vi "ListboxStimulus.vi"(11 "error in (no error)":errorcluster) -> (15 "error out":errorcluster)   [LabVIEW 2016, in "DronaTest.lvlib"]
uses:
  DronaTest.lvlib
  APIs/Stimulus/ControlValue/SetValueAuto.vi
  APIs/Stimulus/ControlValue/Controls/Listbox/SetValueByItemIndex.vi
  APIs/Assert/AssertControlValue/Equal.vi
  APIs/Stimulus/ControlValue/Controls/Listbox/SetValueByItemName.vi
  APIs/Stimulus/VI/CloseVI.vi
  <vilib>/addons/_JKI Toolkits/Caraya/classes/Test/Test.lvclass
  Drona.lvlib
  <vilib>/SLL Toolkit/SLL Debug/SLL Debug.lvlib
  APIs/Stimulus/ControlValue/ControlValue.lvlib
  APIs/Assert/AssertControlValue/AssertControlValue.lvlib
  APIs/Stimulus/VI/VI.lvlib
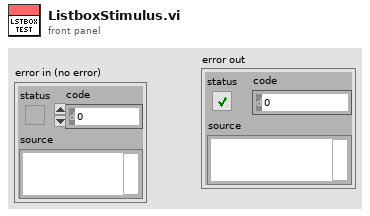
[diagram p1: front panel]
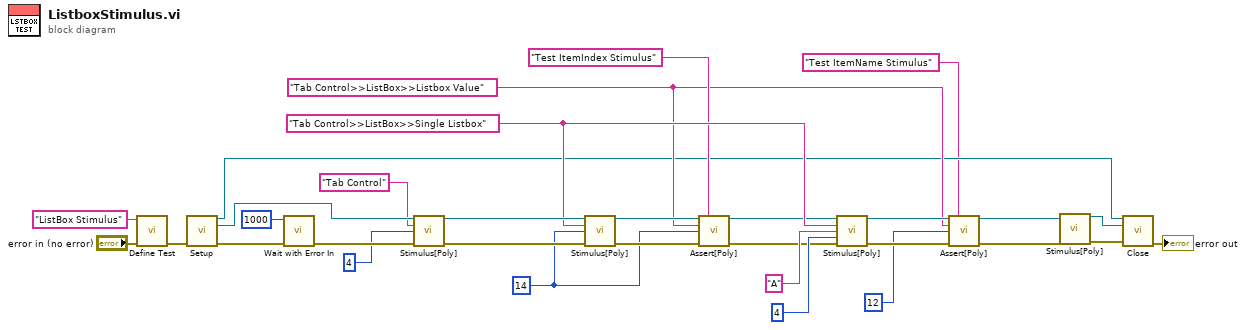
[diagram p0: block diagram]
diagram:
  w8 = "Tab Control>>ListBox>>Listbox Value" ("Control Path")
  w14 = 14 ("Item Index")
  w17 = "Tab Control>>ListBox>>Single Listbox" ("Control Path")
  n1 = call <vilib>:"Define Test.vi"("error in (no error)"="error in (no error)", "Label (VI Title)"="ListBox Stimulus") -> ("error out"=w30:errorcluster)  [unwired: 9 in]
  n2 = call "Setup.vi"("error in"=w30) -> ("Application Ref"=w2:refnum<vi>, "VI Reference Out"=w24:refnum<vi>, "error out"=w29:errorcluster)  [unwired: 12 in]
  n3 = call <vilib>:"Wait with Error In.vi"("error in (no error)"=w29, "milliseconds to wait"=u32 1000) -> ("error out"=w26:errorcluster)  [unwired: 9 in]
  n4 = call-poly "Stimulus[Poly].vi"("VI Reference In"=w24, "Control Path"="Tab Control", "Value (Signaling)"=4, "error in"=w26) -> ("VI Reference Out"=w18:refnum<vi>, "error out"=w25:errorcluster)  [unwired: 10 in]
  n5 = call-poly "Stimulus[Poly].vi"("VI Reference In"=w18, "Control Path"=w17, "Item Index"=w14, "Error In"=w25) -> ("VI Reference Out"=w15:refnum<vi>, "Error Out"=w16:errorcluster)  [unwired: 10 in]
  n6 = call-poly "Assert[Poly].vi"("VI Reference In"=w15, "Test Label"="Test ItemIndex Stimulus", "Control Path"=w8, "Control Value"=w14, "Error In"=w16) -> ("VI Reference Out"=w11:refnum<vi>, "Error Out"=w12:errorcluster)  [unwired: 9 in]
  n7 = call-poly "Stimulus[Poly].vi"("VI Reference In"=w11, "Control Path"=w17, "Item Name"="A", "Occurance"=4, "Error In"=w12) -> ("VI Reference Out"=w9:refnum<vi>, "Error Out"=w10:errorcluster)  [unwired: 9 in]
  n8 = call-poly "Assert[Poly].vi"("VI Reference In"=w9, "Test Label"="Test ItemName Stimulus", "Control Path"=w8, "Control Value"=12 ("Occurance"), "Error In"=w10) -> ("VI Reference Out"=w3:refnum<vi>, "Error Out"=w4:errorcluster)  [unwired: 9 in]
  n9 = call-poly "Stimulus[Poly].vi"("VI Reference In"=w3, "error in"=w4) -> ("VI Reference Out"=w6:refnum<vi>, "error out"=w5:errorcluster)  [unwired: 12 in]
  n10 = call "Close.vi"("Application Ref"=w2, "VI Reference"=w6, "error in"=w5) -> ("error out"=→"error out":errorcluster)  [unwired: 12 in]
